vi "Put-Ball_Api.vi"(7 "執行補值、校正?":bool, 8 "Error In":errorcluster, 9 "輸出位移距離2":dbl[](array[numeric]), 11 "輸出移動距離":dbl[](array[numeric])) -> (0 "Error Out":errorcluster)   [LabVIEW 2019]
uses:
  Variable/Go-Home.vi
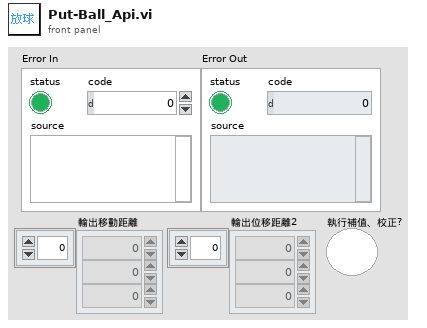
[diagram p1: front panel]
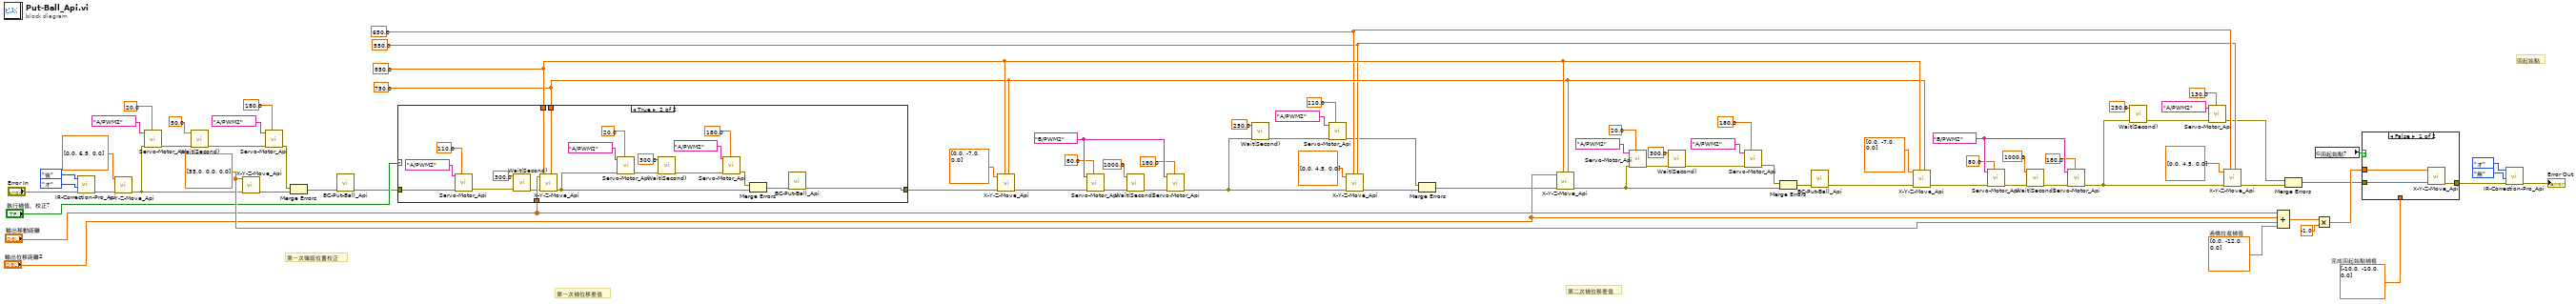
[diagram p0: block diagram]
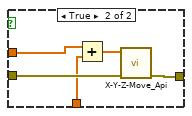
[diagram p3: hidden frame]
diagram:
  w49 = 550.0 ("加速度")
  w50 = 650.0 ("最高速")
  w59 = dbl[] [-10.0, -10.0, 0.0]  # 完成回起始點補植
  w51 = 750.0 ("加速度")
  w52 = 850.0 ("最高速")
  w67 = dbl[] [0.0, -12.0, 0.0]  # 過橋拉進補值
  w78 = tag "B/PWM2" ("伺服馬達角位")
  w81 = tag "B/PWM2" ("伺服馬達角位")
  w56 = dbl[] [55.0, 0.0, 0.0] ("X-Y-Z移動")
  # "回起始點"
  # "第二次補位移差值"
  # "第一次補位移差值"
  # "第一次確認位置校正"
  n1 = call "IR-Correction-Pro_Api.vi"("Error In"="Error In", "副邊校正"=enum16{"前", "後", "オ", "右", "無"}."オ", "主編校正"=enum16{"前", "後", "オ", "右", "無"}."後") -> ("Error Out"=w3:errorcluster)  [unwired: 8 in]
  n2 = call "X-Y-Z-Move_Api.vi"("Error In"=w3, "X-Y-Z移動"=dbl[] [0.0, 6.5, 0.0]) -> ("Error Out"=w22:errorcluster)  [unwired: 8 in, 1 out]
  n3 = call "Servo-Motor_Api.vi"("角度"=20.0, "Error In"=w22, "伺服馬達角位"=tag "A/PWM2") -> ("Error Out"=w28:errorcluster)  [unwired: 8 in]
  n4 = call "Wait(Second).vi"("Error In"=w28, "等待秒數(3000毫秒)"=50.0) -> ("Error Out"=w27:errorcluster)  [unwired: 9 in]
  n5 = call "X-Y-Z-Move_Api.vi"("Error In"=w22, "X-Y-Z移動"=w56) -> ("Error Out"=w48:errorcluster)  [unwired: 8 in, 1 out]
  n6 = call "Servo-Motor_Api.vi"("角度"=180.0, "Error In"=w27, "伺服馬達角位"=tag "A/PWM2") -> ("Error Out"=w21:errorcluster)  [unwired: 8 in]
  n7 = Merge Errors(w21, w48) -> (w23:errorcluster)
  n8 = call "BC-Put-Ball_Api.vi"("Error In"=w23) -> ("Error Out"=w46:errorcluster)  [unwired: 10 in]
  n9 = case shown="True" "執行補值、校正?" {
    tunnel: "輸出移動距離" -> [_ w102]
    tunnel: w46 -> [w82 w84]
    tunnel: [w82 w92] -> w47
    tunnel: w52 -> [_ w99]
    tunnel: w51 -> [_ w93]
    frame False {
    }
    frame True {
      n10 = call "Servo-Motor_Api.vi"("角度"=110.0, "Error In"=w84, "伺服馬達角位"=tag "A/PWM2") -> ("Error Out"=w88:errorcluster)  [unwired: 8 in]
      n11 = call "Wait(Second).vi"("Error In"=w88, "等待秒數(3000毫秒)"=300.0) -> ("Error Out"=w83:errorcluster)  [unwired: 9 in]
      n12 = call "X-Y-Z-Move_Api.vi"("加速度"=w93, "最高速"=w99, "Error In"=w83, "X-Y-Z移動"=w102) -> ("Error Out"=w100:errorcluster)  [unwired: 6 in, 1 out]
      n13 = call "Servo-Motor_Api.vi"("角度"=20.0, "Error In"=w100, "伺服馬達角位"=tag "A/PWM2") -> ("Error Out"=w90:errorcluster)  [unwired: 8 in]
      n14 = call "Wait(Second).vi"("Error In"=w90, "等待秒數(3000毫秒)"=300.0) -> ("Error Out"=w89:errorcluster)  [unwired: 9 in]
      n15 = call "Servo-Motor_Api.vi"("角度"=180.0, "Error In"=w89, "伺服馬達角位"=tag "A/PWM2") -> ("Error Out"=w96:errorcluster)  [unwired: 8 in]
      n16 = Merge Errors(w96, w100) -> (w98:errorcluster)
      n17 = call "BC-Put-Ball_Api.vi"("Error In"=w98) -> ("Error Out"=w92:errorcluster)  [unwired: 10 in]
    }
  }
  n18 = call "X-Y-Z-Move_Api.vi"("加速度"=w51, "最高速"=w52, "Error In"=w47, "X-Y-Z移動"=dbl[] [0.0, -7.0, 0.0]) -> ("Error Out"=w69:errorcluster)  [unwired: 6 in, 1 out]
  n19 = call "Servo-Motor_Api.vi"("角度"=80.0, "Error In"=w69, "伺服馬達角位"=w81) -> ("Error Out"=w80:errorcluster)  [unwired: 8 in]
  n20 = call "Wait(Second).vi"("Error In"=w80, "等待秒數(3000毫秒)"=1000.0) -> ("Error Out"=w79:errorcluster)  [unwired: 9 in]
  n21 = call "Servo-Motor_Api.vi"("角度"=180.0, "Error In"=w79, "伺服馬達角位"=w81) -> ("Error Out"=w13:errorcluster)  [unwired: 8 in]
  n22 = call "Wait(Second).vi"("Error In"=w13, "等待秒數(3000毫秒)"=250.0) -> ("Error Out"=w12:errorcluster)  [unwired: 9 in]
  n23 = call "Servo-Motor_Api.vi"("角度"=110.0, "Error In"=w12, "伺服馬達角位"=tag "A/PWM2") -> ("Error Out"=w35:errorcluster)  [unwired: 8 in]
  n24 = call "X-Y-Z-Move_Api.vi"("加速度"=w49, "最高速"=w50, "Error In"=w13, "X-Y-Z移動"=dbl[] [0.0, 4.5, 0.0]) -> ("Error Out"=w34:errorcluster)  [unwired: 6 in, 1 out]
  n25 = Merge Errors(w35, w34) -> (w33:errorcluster)
  n26 = call "X-Y-Z-Move_Api.vi"("加速度"=w51, "最高速"=w52, "Error In"=w33, "X-Y-Z移動"="輸出位移距離2") -> ("Error Out"=w65:errorcluster)  [unwired: 6 in, 1 out]
  n27 = call "Servo-Motor_Api.vi"("角度"=20.0, "Error In"=w65, "伺服馬達角位"=tag "A/PWM2") -> ("Error Out"=w19:errorcluster)  [unwired: 8 in]
  n28 = call "Wait(Second).vi"("Error In"=w19, "等待秒數(3000毫秒)"=300.0) -> ("Error Out"=w18:errorcluster)  [unwired: 9 in]
  n29 = call "Servo-Motor_Api.vi"("角度"=180.0, "Error In"=w18, "伺服馬達角位"=tag "A/PWM2") -> ("Error Out"=w60:errorcluster)  [unwired: 8 in]
  n30 = Merge Errors(w60, w65) -> (w62:errorcluster)
  n31 = call "BC-Put-Ball_Api.vi"("Error In"=w62) -> ("Error Out"=w17:errorcluster)  [unwired: 10 in]
  n32 = call "X-Y-Z-Move_Api.vi"("加速度"=w51, "最高速"=w52, "Error In"=w17, "X-Y-Z移動"=dbl[] [0.0, -7.0, 0.0]) -> ("Error Out"=w16:errorcluster)  [unwired: 6 in, 1 out]
  n33 = call "Servo-Motor_Api.vi"("角度"=80.0, "Error In"=w16, "伺服馬達角位"=w78) -> ("Error Out"=w77:errorcluster)  [unwired: 8 in]
  n34 = call "Wait(Second).vi"("Error In"=w77, "等待秒數(3000毫秒)"=1000.0) -> ("Error Out"=w76:errorcluster)  [unwired: 9 in]
  n35 = call "Servo-Motor_Api.vi"("角度"=180.0, "Error In"=w76, "伺服馬達角位"=w78) -> ("Error Out"=w9:errorcluster)  [unwired: 8 in]
  n36 = call "Wait(Second).vi"("Error In"=w9, "等待秒數(3000毫秒)"=250.0) -> ("Error Out"=w10:errorcluster)  [unwired: 9 in]
  n37 = call "Servo-Motor_Api.vi"("角度"=130.0, "Error In"=w10, "伺服馬達角位"=tag "A/PWM2") -> ("Error Out"=w15:errorcluster)  [unwired: 8 in]
  n38 = call "X-Y-Z-Move_Api.vi"("加速度"=w49, "最高速"=w50, "Error In"=w9, "X-Y-Z移動"=dbl[] [0.0, 4.5, 0.0]) -> ("Error Out"=w39:errorcluster)  [unwired: 6 in, 1 out]
  n39 = Compound Arithmetic op=ADD("輸出移動距離", "輸出位移距離2", w56, w67) -> (w75:dbl[])
  n40 = Merge Errors(w15, w39) -> (w38:errorcluster)
  n41 = global read "Go-Home.vi" "回起始點?"() -> (w58:bool)
  n42 = Multiply(x=w75, y=-1.0) -> (x*y=w73:dbl[])
  n43 = case shown="False" w58 {
    tunnel: [w105 w109] -> w8
    tunnel: w73 -> [w104 w107]
    tunnel: w38 -> [w103 w110]
    tunnel: w59 -> [_ w106]
    frame False {
      n44 = call "X-Y-Z-Move_Api.vi"("Error In"=w103, "X-Y-Z移動"=w104) -> ("Error Out"=w105:errorcluster)  [unwired: 8 in, 1 out]
    }
    frame True {
      n45 = Add(x=w107, y=w106) -> (x+y=w108:dbl[])
      n46 = call "X-Y-Z-Move_Api.vi"("Error In"=w110, "X-Y-Z移動"=w108) -> ("Error Out"=w109:errorcluster)  [unwired: 8 in, 1 out]
    }
  }
  n47 = call "IR-Correction-Pro_Api.vi"("Error In"=w8, "副邊校正"=enum16{"前", "後", "オ", "右", "無"}."無", "主編校正"=enum16{"前", "後", "オ", "右", "無"}."オ") -> ("Error Out"=→"Error Out":errorcluster)  [unwired: 8 in]
